vi "TupnOff.vi"(11 "Pump_1AI_1DO_2DI in":refnum<class "Engine_1DI_2DO.lvclass">) -> (3 "Pump_1AI_1DO_2DI out":refnum<class "Engine_1DI_2DO.lvclass">)   [LabVIEW 2019, in "Engine_1DI_2DO.lvclass"]
uses:
  Engine_1DI_2DO.lvclass
  Engine_1DI_2DO.lvclass/Engine_1DI_2DO.ctl
  TypeDef/StatePump.ctl
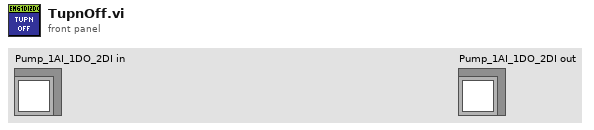
[diagram p1: front panel]
types:
  T1 = typedef "StatePump.ctl" = enum16{"Off", "TupningOn", "On", "TurningOff"}
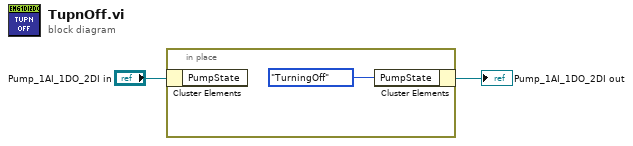
[diagram p0: block diagram]
diagram:
  n1 = in-place {
    n2 = in-place-cluster #1("Pump_1AI_1DO_2DI in") -> ()  [unwired: 1 out]
    n3 = in-place-cluster #1("PumpState"=StatePump."TurningOff") -> (→"Pump_1AI_1DO_2DI out":refnum<class "Engine_1DI_2DO.lvclass">)
  }
